vi "Set Create Temporary Log Files.vi"(8 "error in (no error)":errorcluster, 10 "CreateTemporaryLogFiles":bool, 11 "Data Logging Specification Ref in":T1) -> (0 "error out":errorcluster, 3 "Data Logging Specification Ref out":T1)   [LabVIEW 2020, in "NI_VS Data Logging API.lvlib"]
uses:
  <vilib>/NI VeriStand/Execution/DataLogging/NI_VS Data Logging API.lvlib
  <vilib>/NI VeriStand/Execution/DataLogging/DataLoggingSpecification Ref.ctl
  NationalInstruments.VeriStand.ClientAPI
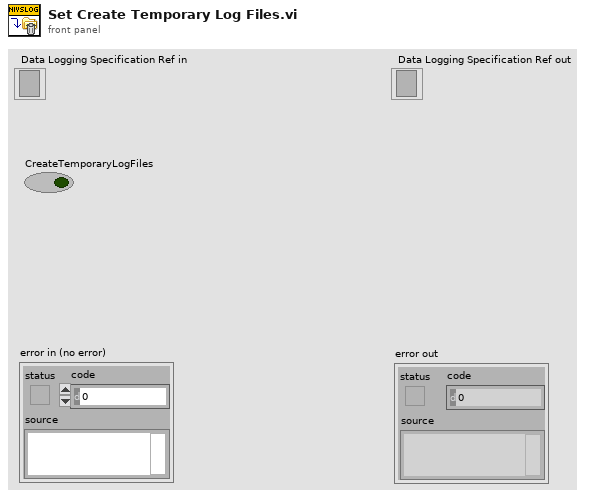
[diagram p1: front panel]
types:
  T1 = typedef "NI_VS Data Logging API.lvlib/DataLoggingSpecification Ref.ctl" = refnum<k24>
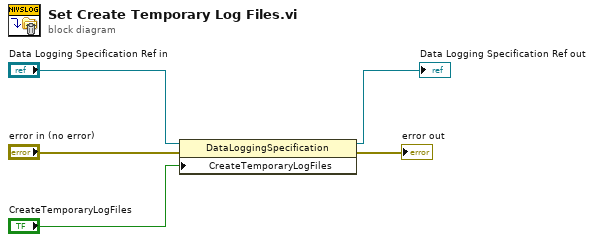
[diagram p0: block diagram]
diagram:
  n1 = property class="DataLoggingSpecification"(reference="Data Logging Specification Ref in", error in="error in (no error)", "CreateTemporaryLogFiles"="CreateTemporaryLogFiles") -> (reference out=→"Data Logging Specification Ref out":T1, error out=→"error out":errorcluster)
